vi "temp_AMTI_meas.vi"() -> ()   [LabVIEW 2015]
uses:
  G 5.lvlib
panel:
  out "ACTUAL DURATION":dbl=1.6
  out "Iteration Time [sec]":dbl=1.6
  in  "ZERO":bool
  out "Output Graph 1":waveform(dbl)[](graph)
  in  "Display Duration [sec] 2":dbl=10.0
  in  "Display Duration [sec]":dbl=10.0
  in  "Gen 5 Displayed 1":i64=1
  in  "stop":bool
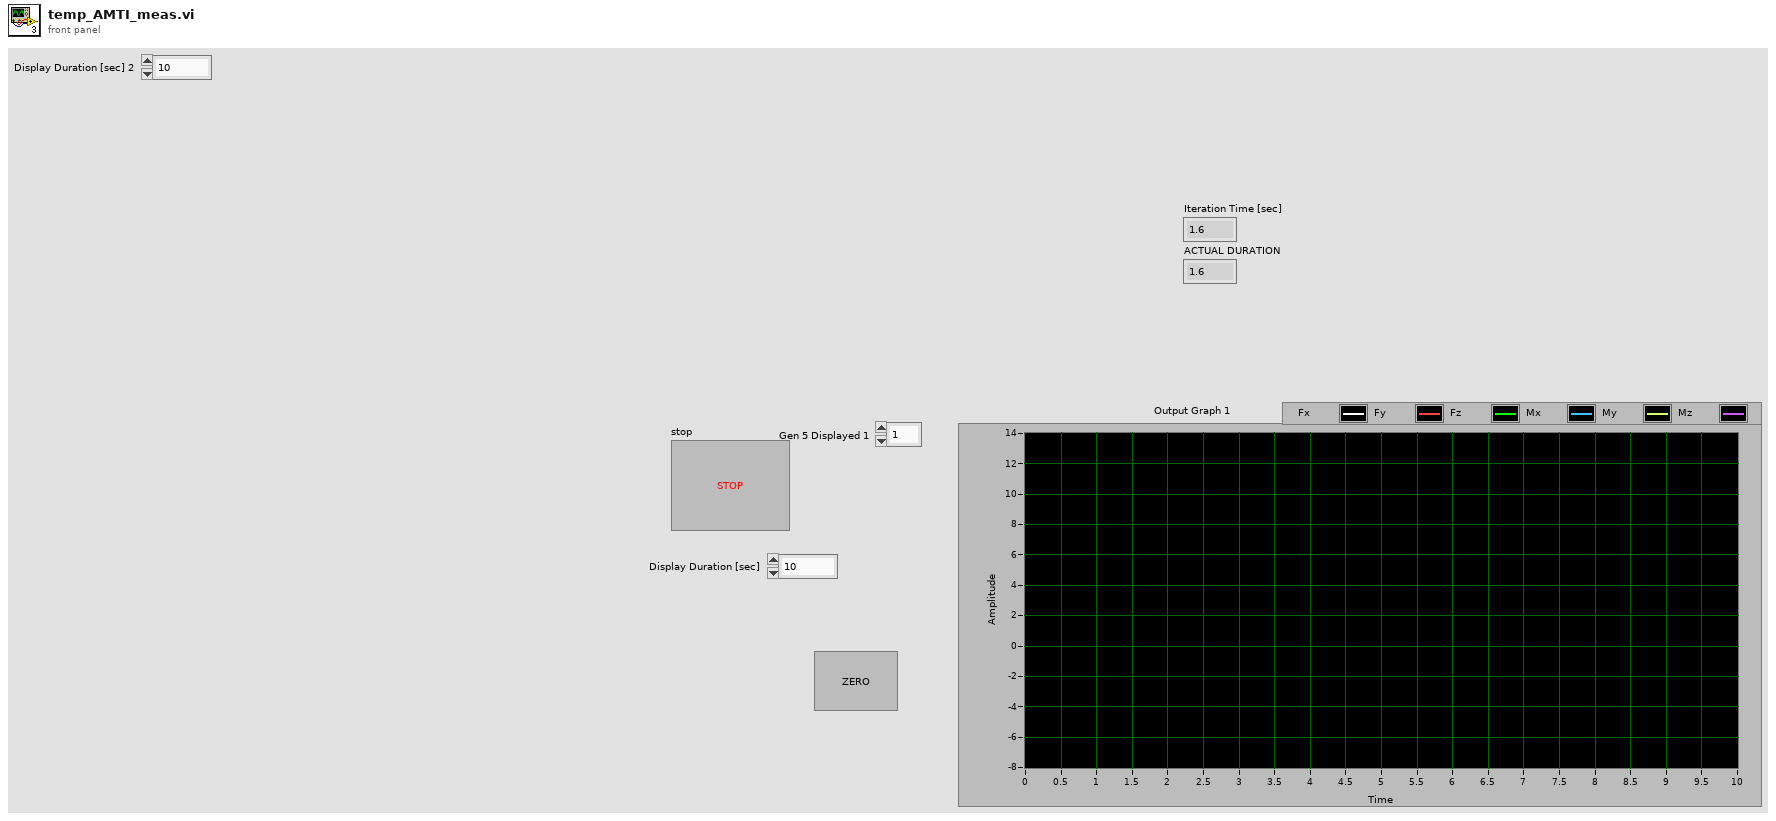
[diagram p1: front panel]
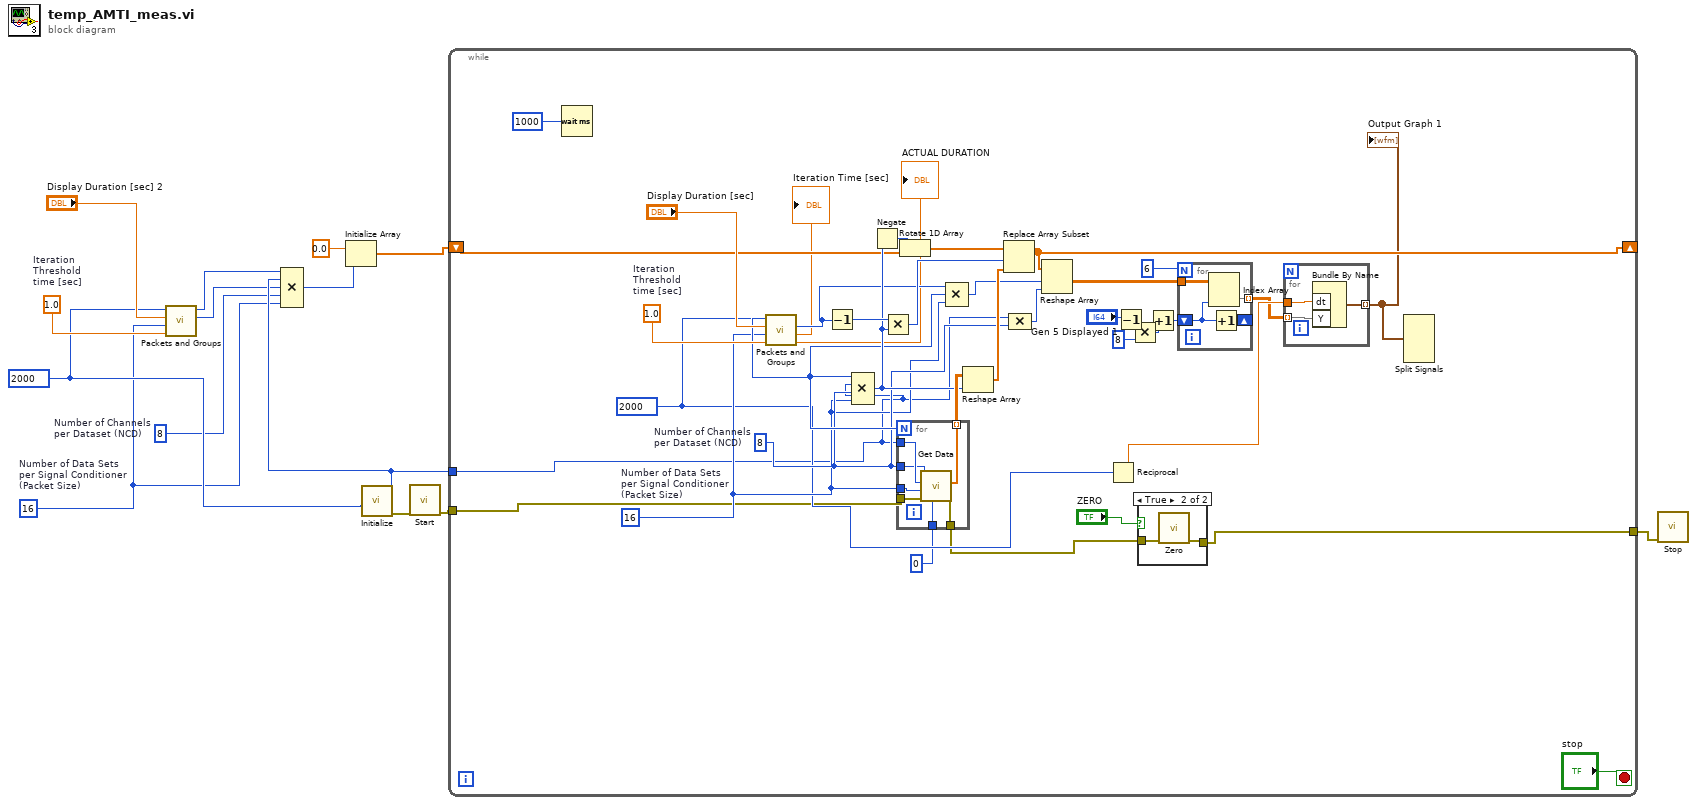
[diagram p0: block diagram]
diagram:
  w5 = i16 2000 items=["10"=10, "15"=15, "20"=20, "25"=25, "30"=30, "40"=40, "45"=45, "50"=50, "60"=60, "75"=75, "80"=80, "90"=90, "100"=100, "120"=120, "125"=125, "150"=150, "180"=180, "200"=200, "225"=225, "240"=240, "250"=250, "300"=300, "360"=360, "400"=400, "450"=450, "500"=500, "600"=600, "800"=800, "900"=900, "1000"=1000, "1200"=1200, "1500"=1500, "1800"=1800, "2000"=2000] ("Acquisition Rate [Hz]")
  w11 = 1.0  # Iteration  Threshold  time [sec]
  w3 = 8  # Number of Channels per Dataset (NCD)
  w2 = 16  # Number of Data Sets  per Signal Conditioner (Packet Size)
  n1 = call "Packets and Groups.vi"("Iteration Treshold Time [sec]"=w11, "Packet Size"=w2, "Duration [sec]"="Display Duration [sec] 2", "Acquisition Rate"=w5) -> ("GROUPS"=w4:i32, "PACKETS"=w7:i32)  [unwired: 4 in, 2 out]
  n2 = call "Initialize.vi"("Acquisition Rate"=w5) -> ("error out"=w13:errorcluster, "Device Count"=w6:i32)  [unwired: 9 in]
  n3 = Compound Arithmetic op=MULTIPLY(w7, w6, w4, w3, w2) -> (w8:i32)
  n4 = Initialize Array(0.0 ("element"), w8) -> (w1:dbl[])
  n5 = call "Start.vi"("error in (no error)"=w13) -> ("error out"=w14:errorcluster)  [unwired: 10 in]
  n6 = while {
    tunnel: w14 -> [w26]
    tunnel: [w18] -> w12
    tunnel: w6 -> [w24]
    shift-right: [w22] -> _
    shift-left: w1 -> [w23]
    stop <- "stop" stop-if-true
    w27 = i16 2000 items=["10"=10, "15"=15, "20"=20, "25"=25, "30"=30, "40"=40, "45"=45, "50"=50, "60"=60, "75"=75, "80"=80, "90"=90, "100"=100, "120"=120, "125"=125, "150"=150, "180"=180, "200"=200, "225"=225, "240"=240, "250"=250, "300"=300, "360"=360, "400"=400, "450"=450, "500"=500, "600"=600, "800"=800, "900"=900, "1000"=1000, "1200"=1200, "1500"=1500, "1800"=1800, "2000"=2000] ("Acquisition Rate [Hz]")
    w33 = 1.0  # Iteration  Threshold  time [sec]
    w29 = 8  # Number of Channels per Dataset (NCD)
    w28 = 16  # Number of Data Sets  per Signal Conditioner (Packet Size)
    n7 = Wait (ms)(milliseconds to wait=u32 1000) -> ()  [unwired: 1 out]
    n8 = call "Packets and Groups.vi"("Iteration Treshold Time [sec]"=w33, "Packet Size"=w28, "Duration [sec]"="Display Duration [sec]", "Acquisition Rate"=w27) -> ("ACTUAL DURATION"=→"ACTUAL DURATION":dbl, "Iteration Time [sec]"=→"Iteration Time [sec]":dbl, "GROUPS"=w31:i32, "PACKETS"=w30:i32)  [unwired: 4 in]
    n9 = Decrement(x=w31) -> (x-1=w47:i32)
    n10 = Compound Arithmetic op=MULTIPLY(w30, w24, w29, w28) -> (w46:i32)
    n11 = Negate(x=w46) -> (-x=w50:i32)
    n12 = Multiply(x=w47, y=w46) -> (x*y=w45:i32)
    n13 = for {
      N: w30 -> [_]
      tunnel: 0 -> [w69]
      tunnel: [w65] -> w19
      tunnel: w24 -> [w66]
      tunnel: w26 -> [w68]
      tunnel: [w67] -> w51 mode=indexing
      tunnel: w28 -> [w64]
      tunnel: w29 -> [w63]
      n14 = call "Get Data.vi"("Iteration"=w69, "error in"=w68, "N_DataSets\nper Gen5"=w64, "Device Count"=w66, "N_Channels\nper Dataset (NCD)"=w63) -> ("error out"=w65:errorcluster, "Data out"=w67:sgl[])  [unwired: 5 in]
    }
    n15 = Rotate 1D Array(1:w23, 2:w50) -> (0:w49:dbl[])
    n16 = Compound Arithmetic op=MULTIPLY(w31, w30, w28) -> (w44:i32)
    n17 = Reshape Array(w51, w46) -> (w48:sgl[])
    n18 = Replace Array Subset(array=w49, new element=w48, index=w45) -> (w22:dbl[])
    n19 = Compound Arithmetic op=MULTIPLY(w24, w29) -> (w43:i32)
    n20 = Reshape Array(w22, w44, w43) -> (w36:dbl[][])
    n21 = Reciprocal(x=w27) -> (1/x=w37:dbl)
    n22 = Decrement(x="Gen 5 Displayed 1") -> (x-1=w40:i64)
    n23 = Multiply(x=w40, y=i64 8) -> (x*y=w38:i64)
    n24 = case shown="True" "ZERO" {
      tunnel: w19 -> [w53 w55]
      tunnel: [w53 w54] -> w18
      frame False {
      }
      frame True {
        n25 = call "Zero.vi"("error in (no error)"=w55) -> ("error out"=w54:errorcluster)  [unwired: 10 in]
      }
    }
    n26 = Increment(x=w38) -> (x+1=w35:i64)
    n27 = for {
      N: 6 -> [_]
      tunnel: w36 -> [w62]
      tunnel: [w61] -> w34 mode=indexing
      shift-right: [w60] -> _
      shift-left: w35 -> [w59]
      n28 = Index Array(array=w62, index (col)=w59) -> (element=w61:dbl[])  [unwired: 1 in]
      n29 = Increment(x=w59) -> (x+1=w60:i64)
    }
    n30 = for {
      tunnel: [w58] -> w21 mode=indexing
      tunnel: w34 -> [w57] mode=indexing
      tunnel: w37 -> [w56]
      n31 = Bundle By Name("dt"=w56, "Y"=w57) -> (w58:waveform(dbl))  [unwired: 1 in]
    }
    "Output Graph 1" <- w21
    n32 = Split Signals(w21) -> ()  [unwired: 6 in, 6 out]
  }
  n33 = call "Stop.vi"("error in (no error)"=w12) -> ()  [unwired: 10 in, 1 out]
